vi "PH_SRDG645.Init.vi"(0 "i ref in":refnum<vi>, 5 "error in":errorcluster) -> (14 "i ref out":refnum<vi>, 19 "error out":errorcluster)   [LabVIEW 2014, in "PH_SRDG645.lvlib"]
doc: "This VI initializes the connection to the hardware and qieries the settings."
uses:
  PH_SRDG645.lvlib
  instr.lib/SRDG645/Stanford Research DG645 - Driver.lvlib
  PH_Basics/PH_Common/PH_Common.lvlib
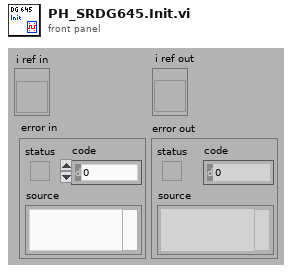
[diagram p1: front panel]
types:
  T1 = typedef "PH_SRDG645.lvlib/PH_SRDG645.i attribute.ctl" = cluster{"GUI Refs":cluster{"Delete":refnum<vi>, "Device Errors":refnum<vi>, "Trigger":refnum<vi>, "Default Name":refnum<vi>, "Firmware Revision":refnum<vi>, "Serial Number":refnum<vi>, "Model":refnum<vi>, "Visa resource name":refnum<vi>}, "Service ID Rate":i32, "Service IDs Channelinfo":i32[], "VISA resource name":refnum<visa-resource-name>, "Device Errors":cluster{"code":i32, "Text":string}[], "Trigger":T2, "Channels":cluster{"T1":T3, "A":T3, "B":T3, "C":T3, "D":T3, "E":T3, "F":T3, "G":T3, "H":T3}, "GUI Refs Channels":refnum<vi>[], "Outputs":cluster{"AB":cluster{"Level Offset [V]":dbl, "Amplitue [V]":dbl, "Polarity":i32}, "CD":cluster{"Level Offset [V]":dbl, "Amplitue [V]":dbl, "Polarity":i32}, "EF":cluster{"Level Offset [V]":dbl, "Amplitue [V]":dbl, "Polarity":i32}, "GH":cluster{"Level Offset [V]":dbl, "Amplitue [V]":dbl, "Polarity":i32}, "T0":cluster{"Level Offset [V]":dbl, "Amplitue [V]":dbl, "Polarity":i32}}, "GUI Refs Outputs":refnum<vi>[], "Serial Number":string, "Firmweare Revision":string, "Model":string}
  T2 = typedef "PH_SRDG645.lvlib/PH_SRDG645.Trigger.ctl" = cluster{"Source":i32, "Rate [Hz]":dbl, "Level [V]":dbl}
  T3 = typedef "PH_SRDG645.lvlib/PH_SRDG645.Channel Settings.ctl" = cluster{"Delay [s]":dbl, "relative to":i32}
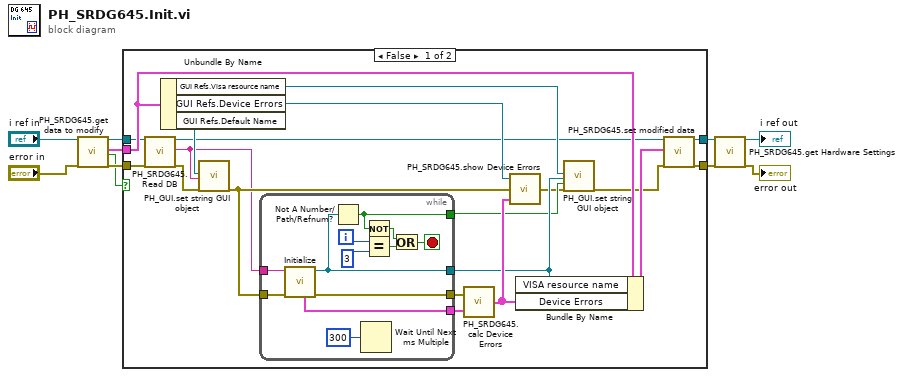
[diagram p0: block diagram]
diagram:
  n1 = call "PH_SRDG645.get data to modify.vi"("i ref in"="i ref in", "error in (no error)"="error in") -> ("i ref out"=w7:refnum<vi>, "i attribute"=w1:T1, "timed out"=w2:bool, "error out"=w4:errorcluster)  [unwired: 14 in]
  n2 = case shown="False" w2 {
    tunnel: w7 -> [w12 w44]
    tunnel: [w30 w43] -> w6
    tunnel: w4 -> [w29 w43]
    tunnel: [w28 w44] -> w3
    tunnel: w1 -> [w26 _]
    frame False {
      n3 = call "PH_SRDG645.Read DB.vi"("i ref in"=w12, "error in"=w29) -> ("i ref out"=w11:refnum<vi>, "Default Name"=w13:string, "error out"=w25:errorcluster)  [unwired: 15 in]
      n4 = Unbundle By Name(w26) -> ("GUI Refs.Visa resource name"=w18:refnum<vi>, "GUI Refs.Device Errors"=w23:refnum<vi>, "GUI Refs.Default Name"=w24:refnum<vi>)
      n5 = call "PH_GUI.set string GUI object.vi"("GUI object Ref"=w24, "Text"=w13, "error in"=w25) -> ("error out"=w20:errorcluster)  [unwired: 16 in]
      n6 = while {
        tunnel: w13 -> [w42]
        tunnel: [w41] -> w22
        tunnel: [w40] -> w21
        tunnel: w20 -> [w39]
        tunnel: [w38] -> w17
        tunnel: [w32] -> w16
        i -> [w37]
        stop <- w34 stop-if-true
        n7 = call "Initialize.vi"("error in (no error)"=w39, "VISA resource name"=w42) -> ("error out"=w41:errorcluster, "VISA resource name out"=w38:refnum<visa-resource-name>, "Device Errors"=w40:cluster{"code":i32, "Text":string}[])  [unwired: 7 in]
        n8 = Not A Number/Path/Refnum?(number/path/refnum=w38) -> (NaN/Path/Refnum?=w32:bool)
        n9 = Wait Until Next ms Multiple(millisecond multiple=u32 300) -> ()  [unwired: 1 out]
        n10 = Not(x=w32) -> (.not. x?=w33:bool)
        n11 = Equal?(x=w37, y=3) -> (x = y?=w35:bool)
        n12 = Or(x=w33, y=w35) -> (x .or. y?=w34:bool)
      }
      n13 = call "PH_SRDG645.calc Device Errors.vi"("Device Errors out"=w21, "SRDG 645 error out"=w22) -> ("calculate Device Errors"=w19:cluster{"code":i32, "Text":string}[])
      n14 = call "PH_SRDG645.show Device Errors.vi"("Device Errors"=w19, "error in"=w20, "Ref Device Errors"=w23) -> ("error out"=w15:errorcluster)
      n15 = Bundle By Name(cluster=w26, "VISA resource name"=w17, "Device Errors"=w19) -> (w27:T1)
      n16 = call "PH_GUI.set string GUI object.vi"("GUI object Ref"=w18, "Text"=w17, "Blinking? (false)"=w16, "error in"=w15) -> ("error out"=w14:errorcluster)  [unwired: 15 in]
      n17 = call "PH_SRDG645.set modified data.vi"("i ref in"=w11, "i attribute"=w27, "error in (no error)"=w14) -> ("i ref out"=w28:refnum<vi>, "error out"=w30:errorcluster)  [unwired: 15 in]
    }
    frame True {
    }
  }
  n18 = call "PH_SRDG645.get Hardware Settings.vi"("i ref in"=w3, "error in"=w6) -> ("i ref out"=→"i ref out":refnum<vi>, "error out"=→"error out":errorcluster)  [unwired: 16 in]
